vi "Set All Controls References to Hash.vi"(8 "error in (no error)":errorcluster, 11 "vi reference (caller)":refnum<vi>) -> (0 "error out":errorcluster, 3 "controls references hash":variant)   [LabVIEW 2013, in "Control Reference.lvlib"]
doc: "Returns all of the controls references with specified VI reference. If leave VI reference unwired, it will use caller's reference."
uses:
  <vilib>/Utility/traverseref.llb/TRef TravTarget.ctl
  Control Reference.lvlib
  <vilib>/Utility/traverseref.llb/VI Scripting - Traverse.lvlib
panel:
  # "set all controls references to hash.vi\nSaves all of the controls references with specified VI reference to hash. If leave VI reference unwired, it will use caller's reference. In the hash, it saves control reference with control label text.\n\nNOTICE -- YOU MUST LEAVE THIS NOTICE IN PLACE.\n\nCopyright (c) 2012, LIANG LIU Shawn.Liu.cn@gmail.com\nAll rights reserved.\n\nRedistribution and use in source and binary forms, with or without modification, are permitted provided that the following conditions are met:\n-Redistributions of source code must retain the above copyright notice, this list of conditions and the following disclaimer.\n-Redistributions in binary form must reproduce the above copyright notice, this list of conditions and the following disclaimer in the documentation and/or other materials provided with the distribution.\n-Neither the name of the eLp nor the names of its contributors may be used to endorse or promote products derived from this software without specific prior written permission.\n\nTHIS SOFTWARE IS PROVIDED BY THE COPYRIGHT HOLDERS AND CONTRIBUTORS \"AS IS\" AND ANY EXPRESS OR IMPLIED WARRANTIES, INCLUDING, BUT NOT LIMITED TO, THE IMPLIED WARRANTIES OF MERCHANTABILITY AND FITNESS FOR A PARTICULAR PURPOSE ARE DISCLAIMED. IN NO EVENT SHALL THE COPYRIGHT HOLDER OR CONTRIBUTORS BE LIABLE FOR ANY DIRECT, INDIRECT, INCIDENTAL, SPECIAL, EXEMPLARY, OR CONSEQUENTIAL DAMAGES (INCLUDING, BUT NOT LIMITED TO, PROCUREMENT OF SUBSTITUTE GOODS OR SERVICES; LOSS OF USE, DATA, OR PROFITS; OR BUSINESS INTERRUPTION) HOWEVER CAUSED AND ON ANY THEORY OF LIABILITY, WHETHER IN CONTRACT, STRICT LIABILITY, OR TORT (INCLUDING NEGLIGENCE OR OTHERWISE) ARISING IN ANY WAY OUT OF THE USE OF THIS SOFTWARE, EVEN IF ADVISED OF THE POSSIBILITY OF SUCH DAMAGE."
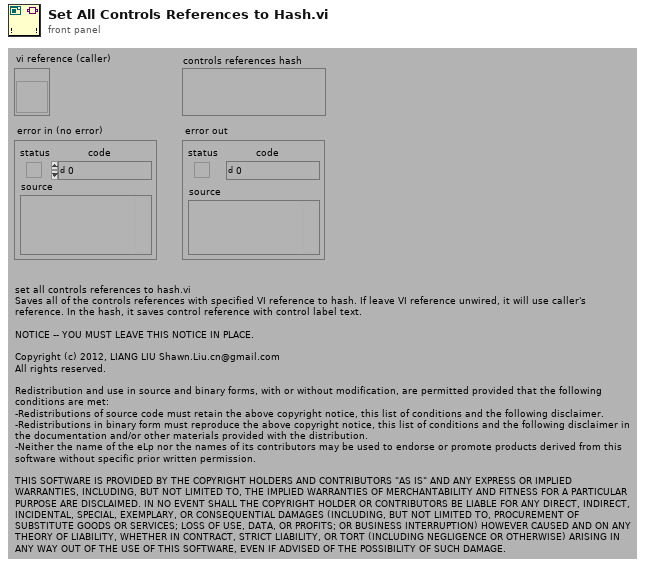
[diagram p1: front panel]
types:
  T1 = typedef "TRef TravTarget.ctl" = enum16{"FP", "BD", "Other"}
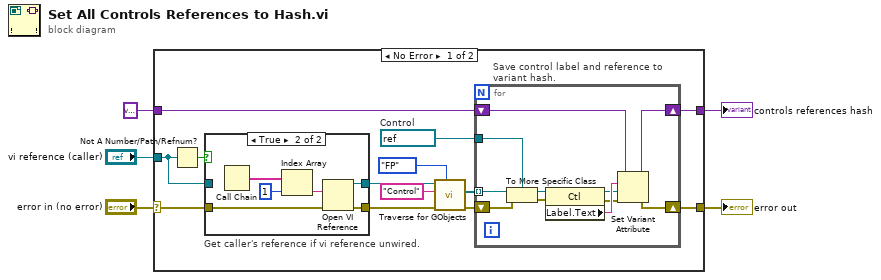
[diagram p0: block diagram]
diagram:
  n1 = case shown="No Error" "error in (no error)" {
    selector: "error in (no error)" -> [w8 w39]
    tunnel: [w15 w38] -> w5
    tunnel: "vi reference (caller)" -> [w13 _]
    tunnel: [w7 w39] -> w2
    tunnel: variant -> [w6 w38]
    frame No Error {
      w11 = refnum<vi> refnum  # Control
      n2 = Not A Number/Path/Refnum?(number/path/refnum=w13) -> (NaN/Path/Refnum?=w14:bool)
      n3 = case "Get caller's reference if vi reference unwired." shown="True" w14 {
        tunnel: [w20 w23] -> w12
        tunnel: w13 -> [w20 _]
        tunnel: [w19 w22] -> w10
        tunnel: w8 -> [w19 w21]
        frame False {
        }
        frame True {
          n4 = Call Chain() -> (call chain=w26:string[])
          n5 = Index Array(array=w26, index=1) -> (element=w24:string)
          n6 = Open VI Reference(vi path=w24, error in (no error)=w21) -> (vi reference=w23:refnum<vi>, error out=w22:errorcluster)  [unwired: 4 out]
        }
      }
      n7 = call <vilib>:"Traverse for GObjects.vi"("Traverse Target"=TRef_TravTarget."FP", "error in (no error)"=w10, "Class Name"="Control", "VI Refnum"=w12) -> ("error out"=w9:errorcluster, "References"=w16:refnum<vi>[])  [unwired: 4 in, 2 out]
      n8 = for "Save control label and reference to\nvariant hash." {
        shift-right: [w31] -> w15
        shift-left: w6 -> [w32]
        tunnel: w16 -> [w37] mode=indexing
        tunnel: w11 -> [w33]
        shift-right: [w27] -> w7
        shift-left: w9 -> [w30]
        n9 = To More Specific Class(target class=w33, reference=w37, error in=w30) -> (specific class reference=w36:refnum<vi>, error out=w29:errorcluster)
        n10 = property class="Ctl"(reference=w36, error in=w29) -> (reference out=w34:refnum<vi>, error out=w28:errorcluster, "Label.Text"=w35:string)
        n11 = Set Variant Attribute(Variant=w32, name=w35, value=w34, error in=w28) -> (Variant out=w31:variant, error out=w27:errorcluster)  [unwired: 1 out]
      }
    }
    frame Error {
    }
  }
  "controls references hash" <- w5
  "error out" <- w2
